vi "STRING SUBSET.vi"() -> ()   [LabVIEW 2019]
panel:
  out "PLACE":string="COIMBATORE"
  out "NAME":string="SURAKSHITH"
  in  "INPUT STRING":string="SURAKSHITH IS FROM COIMBATORE"
  # "STRING SUBSET"
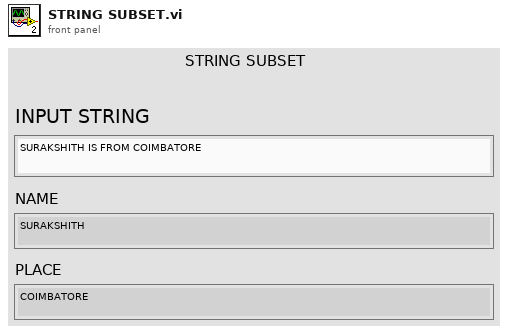
[diagram p1: front panel]
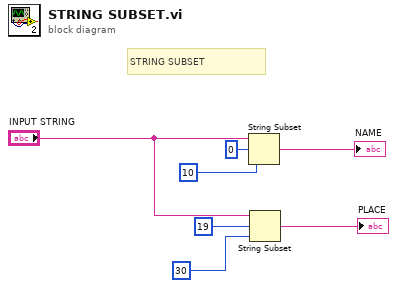
[diagram p0: block diagram]
diagram:
  # "STRING SUBSET"
  n1 = String Subset(string="INPUT STRING", offset (0)=0, length (rest)=10 ("length (rest)")) -> (substring=→"NAME":string)
  n2 = String Subset(string="INPUT STRING", offset (0)=19, length (rest)=30 ("length (rest)")) -> (substring=→"PLACE":string)
